vi "DualMotorSpeed.vi"(4 "Motor 2":string="My Motor RefNum", 6 "Motor 1":string="My Motor RefNum", 9 "Throttle/Speed":dbl, 10 "Run Backward":bool, 11 "Run Forward":bool) -> ()   [LabVIEW 2015, in "hhVI.lvlib"]
uses:
  hhVI.lvlib
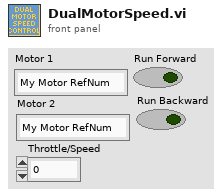
[diagram p1: front panel]
types:
  T1 = typedef "WPI_MotorControlDeviceRef.ctl" = cluster{"DeviceStatus":errorcluster, "Type":T2, "PWM":cluster{"PWM Channel":T3, "DeadBand":T4}, "CAN":cluster{"Device Number":u8, "Control Mode":T5, "Semaphore":T6, "Max Vout":dbl, "TalonSRX Control Mode":T7}, "Invert":bool}
  T2 = typedef "WPI_MotorControlType.ctl" = enum16{"PWM", "CAN", "CANTalonSRX"}
  T3 = typedef "FPGA_DIOPWMChannel.ctl" = enum8{"PWM 0", "PWM 1", "PWM 2", "PWM 3", "PWM 4", "PWM 5", "PWM 6", "PWM 7", "PWM 8", "PWM 9", "PWM MXP 0", "PWM MXP 1", "PWM MXP 2", "PWM MXP 3", "PWM MXP 4", "PWM MXP 5", "PWM MXP 6", "PWM MXP 7", "PWM MXP 8", "PWM MXP 9", "Invalid"}
  T4 = typedef "WPI_PWMDeadband.ctl" = cluster{"Name":string, "maxPositivePwm":i32, "minPositivePwm":i32, "centerPwm":i32, "maxNegativePwm":i32, "minNegativePwm":i32, "angularRange":u16}
  T5 = typedef "WPI_CANJaguar_ControlMode.ctl" = enum8{"Percent VBus", "Current", "Speed", "Position", "Voltage"}
  T6 = typedef "Semaphore RefNum" = refnum<k1>
  T7 = typedef "WPI_CANTalonSRX_APIControlMode.ctl" = enum8{"Percent VBus", "Speed", "Position", "Slave", "Unchanged / Invalid", "Voltage Compensation", "Current", "Motion Profile"}
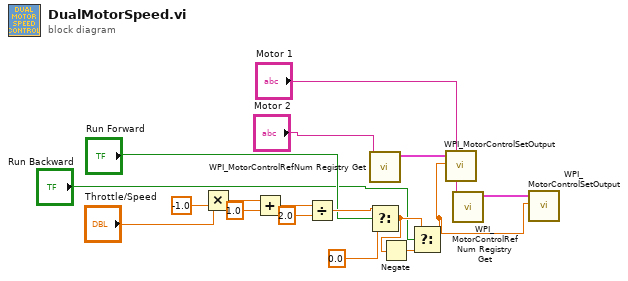
[diagram p0: block diagram]
diagram:
  n1 = Multiply(x="Throttle/Speed", y=-1.0) -> (x*y=w12:dbl)
  n2 = Add(x=w12, y=1.0) -> (x+y=w14:dbl)
  n3 = Divide(x=w14, y=2.0) -> (x/y=w10:dbl)
  n4 = call <vilib>:"WPI_MotorControlRefNum Registry Get.vi"("refnum name"="Motor 2") -> ("MotorControlDevRef"=w17:T1)  [unwired: 9 in, 1 out]
  n5 = Select(t=w10, s="Run Forward", f=0.0) -> (s? t:f=w6:dbl)
  n6 = Negate(x=w6) -> (-x=w7:dbl)
  n7 = Select(t=w6, s="Run Backward", f=w7) -> (s? t:f=w8:dbl)
  n8 = call <vilib>:"WPI_MotorControlSetOutput.vi"("Output"=w8, "MotorControlDevRef"=w17) -> ()  [unwired: 7 in, 3 out]
  n9 = call <vilib>:"WPI_MotorControlRefNum Registry Get.vi"("refnum name"="Motor 1") -> ("MotorControlDevRef"=w9:T1)  [unwired: 9 in, 1 out]
  n10 = call <vilib>:"WPI_MotorControlSetOutput.vi"("Output"=w8, "MotorControlDevRef"=w9) -> ()  [unwired: 7 in, 3 out]
